vi "FTW-Logger-Connect.vi"(5 "Logger Address":string, 11 "error in":errorcluster) -> (4 "FTW Logger Connector":refnum<class "FTW-Logger.lvclass">, 15 "error out":errorcluster)   [LabVIEW 2013, in "FTW-Actor.lvlib" / "FTW-Logger.lvclass"]
doc: "This method launches a Logger Process which is then referred to based on its LoggerID. Normally in a LabVIEW application, an object's methods would adhere to dataflow with the object wired to the method; however, the Logger Process object likely needs to be accessed by many different portions of your application, and for this reason, it is called by reference, where the LoggerID string refers to the logger.\n\nThis method should be called as one of the very first actions in your application to reasonably ensure the buffer of logged events does not overflow. Events that are logged prior to launching the Logger Process with this method are queued, and will be logged once this process begins."
uses:
  FTW-Logger.lvclass
panel:
  # "Inputs"
  # "Outputs"
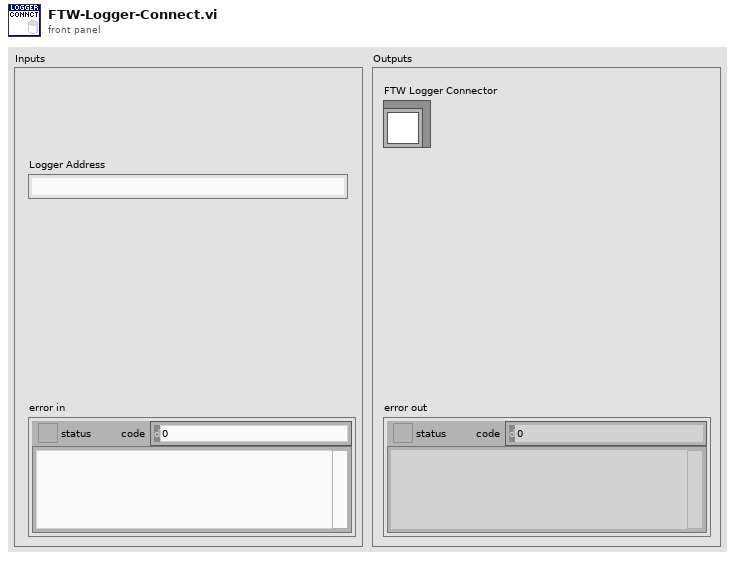
[diagram p1: front panel]
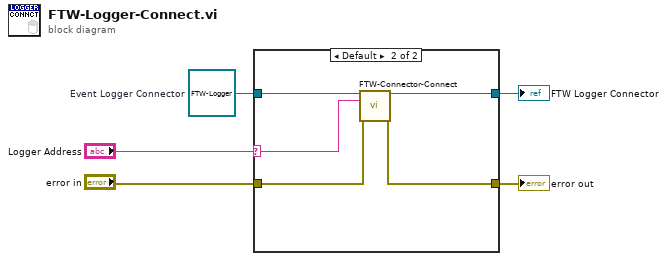
[diagram p0: block diagram]
diagram:
  w2 = refnum<class "FTW-Logger.lvclass"> refnum  # Event Logger Connector
  n1 = case shown="Default" "Logger Address" {
    selector: "Logger Address" -> [_ w8]
    tunnel: [w6 w12] -> w5
    tunnel: "error in" -> [w6 w11]
    tunnel: [w7 w10] -> w3
    tunnel: w2 -> [w7 w9]
    frame "" {
    }
    frame Default {
      n2 = call-dynamic "FTW-Connector-Connect.vi"("FTW Actor Connector Type"=w9, "Instance Inbox Address"=w8, "error in"=w11) -> ("FTW Actor Connector"=w10:refnum<class "FTW-Logger.lvclass">, "error out"=w12:errorcluster)  [unwired: 11 in]
    }
  }
  "error out" <- w5
  "FTW Logger Connector" <- w3
